vi "Page_Source_Add.vi"(4 "ctlReferences":T2, 6 "sourceInclusion":T1, 7 "items to add in":string[](array[string]), 8 "error in (no error)":errorcluster, 9 "send to main dest?":bool, 10 "Project Refnum":refnum<vi>, 11 "AB_Source in":refnum<class "AB_Source.lvclass">) -> (0 "error out":errorcluster, 2 "changed":bool, 3 "AB_Source out":refnum<class "AB_Source.lvclass">, 5 "items to add out":string[](array[string]))   [LabVIEW 2020, in "AB_Source.lvclass"]
uses:
  <vilib>/AppBuilder/AB_Classes/Source/AB_Source.lvclass
  <resource>/Framework/Providers/Builds/AppBuilder/AB_UI_Page_Source_Files_References.ctl
  <vilib>/AppBuilder/AB_Source_Inclusion.ctl
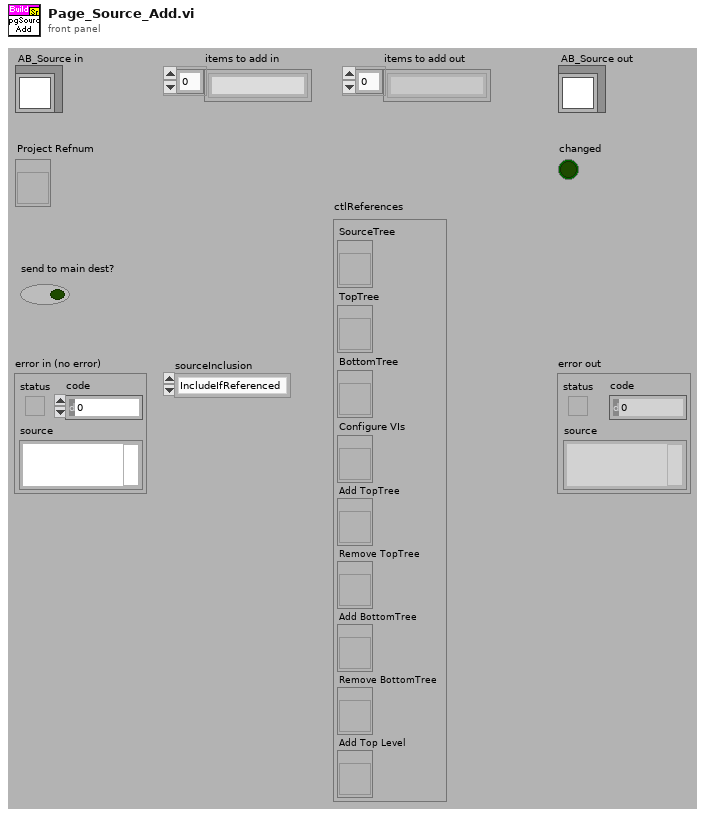
[diagram p1: front panel]
types:
  T1 = typedef "AB_Source_Inclusion.ctl" = enum16{"IncludeIfReferenced", "Include", "Exclude", "TopLevel"}
  T2 = typedef "AB_UI_Page_Source_Files_References.ctl" = cluster{"SourceTree":refnum<vi>, "TopTree":refnum<vi>, "BottomTree":refnum<vi>, "Configure VIs":refnum<vi>, "Add TopTree":refnum<vi>, "Remove TopTree":refnum<vi>, "Add BottomTree":refnum<vi>, "Remove BottomTree":refnum<vi>, "Add Top Level":refnum<vi>}
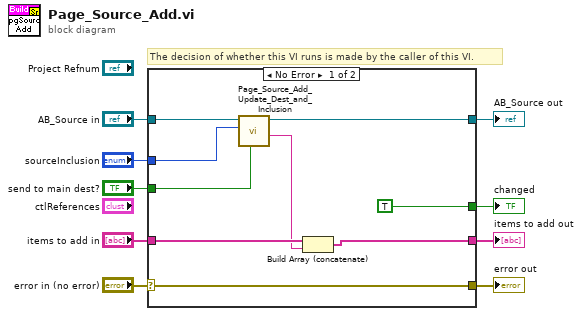
[diagram p0: block diagram]
diagram:
  # "The decision of whether this VI runs is made by the caller of this VI."
  n1 = case shown="No Error" "error in (no error)" {
    selector: "error in (no error)" -> [w18 w20]
    tunnel: [w18 w20] -> w8
    tunnel: [w17 w19] -> w6
    tunnel: "AB_Source in" -> [w16 w19]
    tunnel: [TRUE _] -> w5
    tunnel: "send to main dest?" -> [w11 _]
    tunnel: "items to add in" -> [w14 _]
    tunnel: [w13 _] -> w2
    tunnel: "sourceInclusion" -> [w10 _]
    frame No Error {
      n2 = call <vilib>:"Page_Source_Add_Update_Dest_and_Inclusion.vi"("send to main destination?"=w11, "Inclusion"=w10, "AB_Source_VI in"=w16) -> ("itemID"=w12:string, "AB_Source_VI out"=w17:refnum<class "AB_Source.lvclass">)  [unwired: 6 in, 1 out]
      n3 = Build Array (concatenate)(w14, w12) -> (w13:string[])
    }
    frame Error {
    }
  }
  "error out" <- w8
  "AB_Source out" <- w6
  "changed" <- w5
  "items to add out" <- w2
